vi "HT.vi"(7 "Auto":bool, 8 "On":bool, 9 "x":dbl, 10 "SP":dbl, 11 "Bool Refnum":refnum<vi>) -> (3 "s? t:f":bool)   [LabVIEW 2013]
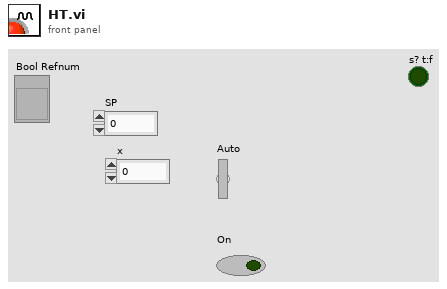
[diagram p1: front panel]
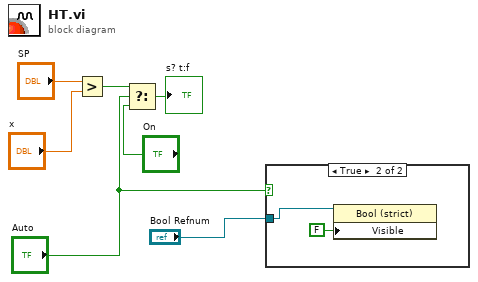
[diagram p0: block diagram]
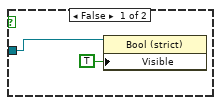
[diagram p2: hidden frame]
diagram:
  n1 = Greater?(x="SP", y="x") -> (0:w5:bool)
  n2 = Select(t=w5, s="Auto", f="On") -> (s? t:f=→"s? t:f":bool)
  n3 = case shown="True" "Auto" {
    tunnel: "Bool Refnum" -> [w9 w11]
    frame False {
      n4 = property class="Bool (strict)"(reference=w9, "Visible"=TRUE) -> ()  [unwired: 1 in, 2 out]
    }
    frame True {
      n5 = property class="Bool (strict)"(reference=w11, "Visible"=FALSE) -> ()  [unwired: 1 in, 2 out]
    }
  }
